vi "Sam_CombineHits.vi"(6 "Delays":T1, 9 "run name":string, 10 "raw files":string[](array[string]), 11 "raw path":path) -> (2 "Data":waveform(dbl)[](array[waveform]), 3 "dt bad?":bool)   [LabVIEW 2022 SP3]
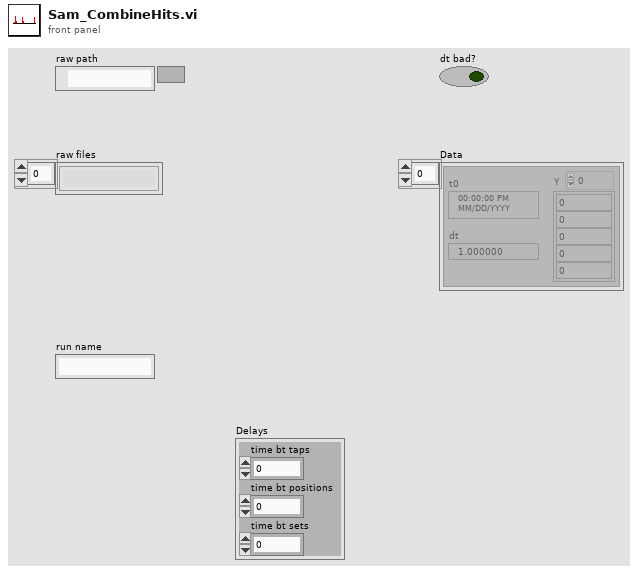
[diagram p1: front panel]
types:
  T1 = cluster{"time bt taps":dbl, "time bt positions":dbl, "time bt sets":dbl}
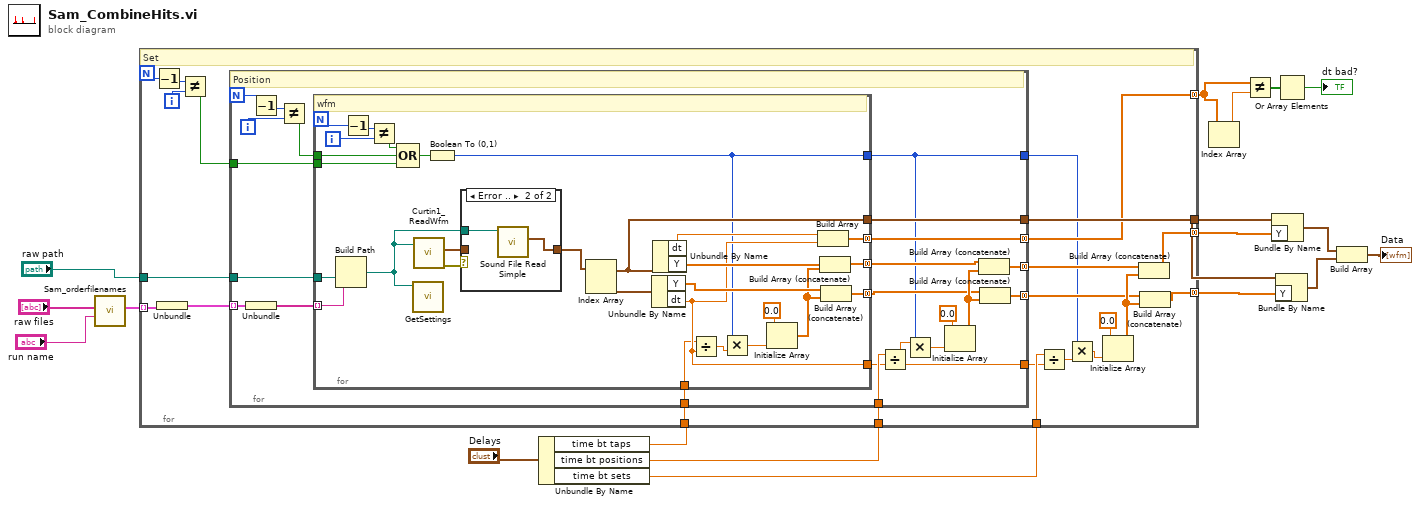
[diagram p0: block diagram]
diagram:
  n1 = call "Sam_orderfilenames.vi"("Original name"="run name", "filenames"="raw files") -> ("Array 3"=w3:cluster{cluster{string[]}[]}[])  [unwired: 9 in]
  n2 = Unbundle By Name("Delays") -> ("time bt taps"=w16:dbl, "time bt positions"=w17:dbl, "time bt sets"=w18:dbl)
  n3 = for {
    N -> [w25]
    tunnel: "raw path" -> [w40]
    tunnel: w3 -> [w39] mode=indexing
    tunnel: w17 -> [w37]
    tunnel: [w36] -> w4
    tunnel: [w31] -> w5 mode=concatenating
    tunnel: [w30] -> w6 mode=concatenating
    tunnel: w18 -> [w29]
    tunnel: [w27] -> w8 mode=concatenating
    tunnel: w16 -> [w26]
    i -> [w23]
    # "Set"
    n4 = Decrement(x=w25) -> (x-1=w24:i32)
    n5 = Unbundle(w39) -> (w38:cluster{string[]}[])
    n6 = Not Equal?(x=w24, y=w23) -> (x != y?=w22:bool)
    n7 = for {
      N -> [w47]
      tunnel: w40 -> [w62]
      tunnel: w38 -> [w61] mode=indexing
      tunnel: w37 -> [w58]
      tunnel: [w57] -> w36
      tunnel: [w53] -> w33 mode=concatenating
      tunnel: [w52] -> w32 mode=concatenating
      tunnel: [w51] -> w28
      tunnel: [w50] -> w27 mode=concatenating
      tunnel: w26 -> [w49]
      tunnel: w22 -> [w44]
      tunnel: [w41] -> w21
      i -> [w46]
      # "Position"
      n8 = Unbundle(w61) -> (w60:string[])
      n9 = Decrement(x=w47) -> (x-1=w48:i32)
      n10 = Not Equal?(x=w48, y=w46) -> (x != y?=w45:bool)
      n11 = for {
        N -> [w71]
        tunnel: [w77] -> w56 mode=concatenating
        tunnel: [w80] -> w54 mode=concatenating
        tunnel: [w86] -> w57
        tunnel: w62 -> [w85]
        tunnel: w60 -> [w83] mode=indexing
        tunnel: [w75] -> w51
        tunnel: [w74] -> w50 mode=concatenating
        tunnel: w49 -> [w73]
        tunnel: w45 -> [w68]
        tunnel: w44 -> [w67]
        tunnel: [w63] -> w41
        i -> [w70]
        # "wfm"
        n12 = Build Path(base path=w85, name or relative path=w83) -> (appended path=w84:path)
        n13 = Decrement(x=w71) -> (x-1=w72:i32)
        n14 = Not Equal?(x=w72, y=w70) -> (x != y?=w69:bool)
        n15 = Compound Arithmetic op=OR(w69, w68, w67) -> (w66:bool)
        n16 = call "GetSettings.vi"("wavform file"=w84) -> ()  [unwired: 9 in, 2 out]
        n17 = call "Curtin1_ReadWfm.vi"("appended path"=w84) -> ("error out"=w90:errorcluster, "all waveforms in record"=w89:waveform(dbl)[])  [unwired: 9 in]
        n18 = Boolean To (0,1)(Boolean=w66) -> (0, 1=w63:i16)
        n19 = case shown="Error .." w90 {
          tunnel: w84 -> [_ w93]
          tunnel: w89 -> [w91 _]
          tunnel: [w91 w92] -> w88
          frame No Error {
          }
          frame Error {
            n20 = call <vilib>:"Sound File Read Simple.vi"("path"=w93) -> ("data"=w92:waveform(dbl)[])  [unwired: 7 in, 3 out]
          }
        }
        n21 = Index Array(array=w88) -> (element #1=w86:waveform(dbl), element #2=w87:waveform(dbl))  [unwired: 2 in]
        n22 = Unbundle By Name(w87) -> ("Y"=w81:dbl[], "dt"=w75:dbl)
        n23 = Unbundle By Name(w86) -> ("dt"=w76:dbl, "Y"=w79:dbl[])
        n24 = Divide(x=w73, y=w75) -> (x/y=w65:dbl)
        n25 = Multiply(x=w63, y=w65) -> (x*y=w64:dbl)
        n26 = Initialize Array(0.0 ("element"), w64) -> (w78:dbl[])
        n27 = Build Array(w76, w75) -> (w74:dbl[])
        n28 = Build Array (concatenate)(w79, w78) -> (w77:dbl[])
        n29 = Build Array (concatenate)(w81, w78) -> (w80:dbl[])
      }
      n30 = Divide(x=w58, y=w51) -> (x/y=w43:dbl)
      n31 = Multiply(x=w43, y=w41) -> (x*y=w42:dbl)
      n32 = Initialize Array(0.0 ("element"), w42) -> (w55:dbl[])
      n33 = Build Array (concatenate)(w56, w55) -> (w53:dbl[])
      n34 = Build Array (concatenate)(w54, w55) -> (w52:dbl[])
    }
    n35 = Divide(x=w29, y=w28) -> (x/y=w20:dbl)
    n36 = Multiply(x=w21, y=w20) -> (x*y=w19:dbl)
    n37 = Initialize Array(0.0 ("element"), w19) -> (w35:dbl[])
    n38 = Build Array (concatenate)(w33, w35) -> (w31:dbl[])
    n39 = Build Array (concatenate)(w32, w35) -> (w30:dbl[])
  }
  n40 = Index Array(array=w8) -> (element=w7:dbl)  [unwired: 1 in]
  n41 = Not Equal?(x=w8, y=w7) -> (x != y?=w9:bool[])
  n42 = Bundle By Name(cluster=w4, "Y"=w5) -> (w13:waveform(dbl))
  n43 = Bundle By Name(cluster=w4, "Y"=w6) -> (w12:waveform(dbl))
  n44 = Or Array Elements(Boolean array=w9) -> (logical OR=→"dt bad?":bool)
  n45 = Build Array(w13, w12) -> (→"Data":waveform(dbl)[])
